vi "WS2812 Open.vi"(8 "Error In":errorcluster, 9 "Data Channel":u8, 10 "Number of LEDs":u16, 11 "LINX Device Config":T1) -> (0 "Error Out":errorcluster, 3 "LINX Device Config":T1)   [LabVIEW 2020, in "LMH-LINX.lvlib" / "Device.lvlib"]
uses:
  Device.lvlib
  Type Defs/LINX Device Config.ctl
  Type Defs/Interface.ctl
  Type Defs/TCP Config.ctl
  Type Defs/Channels.ctl
  Type Defs/Error Type.ctl
  LMH-LINX.lvlib
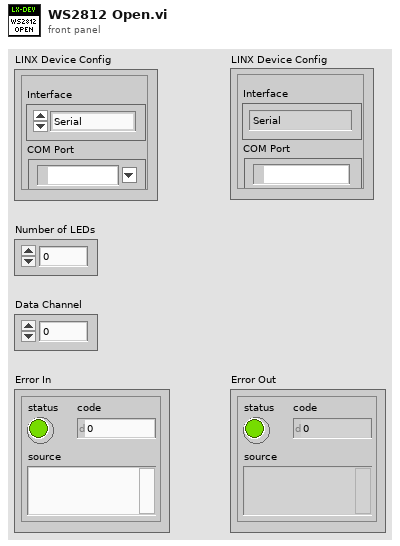
[diagram p1: front panel]
types:
  T1 = typedef "LMH-LINX.lvlib/Device.lvlib/LINX Device Config.ctl" = cluster{"Interface":T2, "COM Port":refnum<visa-resource-name>, "TCP Configuration":T3, "Device Family":u8, "Device ID":u8, "Device Name":string, "TCP Ref":refnum<k5>, "Channels":T4}
  T2 = typedef "LMH-LINX.lvlib/Interface.ctl" = enum16{"Serial", "TCP"}
  T3 = typedef "LMH-LINX.lvlib/Device.lvlib/TCP Config.ctl" = cluster{"IP Address":string, "Port":u16}
  T4 = typedef "LMH-LINX.lvlib/Channels.ctl" = cluster{"DI":u8[], "DO":u8[], "AI":u8[], "AO":u8[], "PWM":u8[], "QE":u8[], "UART":u8[], "I2C 2":u8[], "SPI":u8[], "CAN":u8[], "Servo":u8[], "AI Ref (V)":dbl, "AI Resolution (Bits)":u8, "AO Ref (V)":dbl, "AO Resolution (Bits)":u8}
  T5 = typedef "LMH-LINX.lvlib/Error Type.ctl" = enum16{"Unknown", "Timeout", "Corrupt Return Packet", "Unable To Connect", "Command Not Supported", "Channel DNE", "Invalid COM Config", "Firmware Version Mismatch", "myRIO Support", "CMD Specific Error", "Local IO Not Supported"}
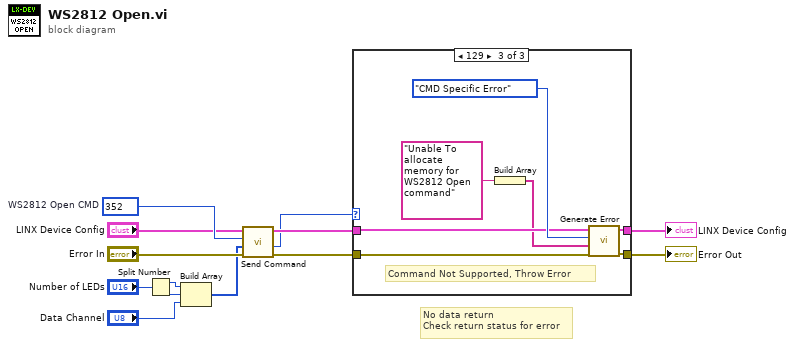
[diagram p0: block diagram]
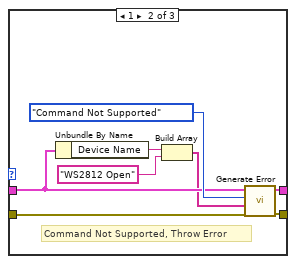
[diagram p3: hidden frame]
diagram:
  w13 = u16 352  # WS2812 Open CMD
  # "No data return\nCheck return status for error"
  n1 = Split Number(x="Number of LEDs") -> (hi(x)=w4:u8, lo(x)=w3:u8)
  n2 = Build Array(w4, w3, "Data Channel") -> (w1:u8[])
  n3 = call "Send Command.vi"("Error In"="Error In", "ARGS"=w1, "CMD"=w13, "LINX Device Config"="LINX Device Config") -> ("Error Out"=w10:errorcluster, "Status"=w8:u8, "LINX Device Config"=w9:T1)  [unwired: 4 in, 1 out]
  n4 = case shown="129" w8 {
    tunnel: [w15 w21 w28] -> w12
    tunnel: w9 -> [w15 w17 w26]
    tunnel: [w14 w22 w29] -> w11
    tunnel: w10 -> [w14 w23 w30]
    frame 0, Default {
      # "Status OK"
    }
    frame 1 {
      # "Command Not Supported, Throw Error"
      n5 = Unbundle By Name(w17) -> ("Device Name"=w19:string)
      n6 = Build Array(w19, "WS2812 Open") -> (w16:string[])
      n7 = call "Generate Error.vi"("Error In"=w23, "Arguments"=w16, "Error Type"=Error_Type."Command Not Supported", "LINX Device Config"=w17) -> ("Error Out"=w22:errorcluster, "Dup LINX Device Config"=w21:T1)  [unwired: 6 in]
    }
    frame 129 {
      # "Command Not Supported, Throw Error"
      n8 = Build Array("Unable To allocate memory for WS2812 Open command") -> (w24:string[])
      n9 = call "Generate Error.vi"("Error In"=w30, "Arguments"=w24, "Error Type"=Error_Type."CMD Specific Error", "LINX Device Config"=w26) -> ("Error Out"=w29:errorcluster, "Dup LINX Device Config"=w28:T1)  [unwired: 6 in]
    }
  }
  "Error Out" <- w11
  "LINX Device Config" <- w12
